vi "Initialize Instrument.vi"(8 "error in (no error)":errorcluster, 10 "Reset":bool, 11 "E3631A in":refnum<class "E3631A.lvclass">) -> (0 "error out":errorcluster, 3 "E3631A out":refnum<class "E3631A.lvclass">)   [LabVIEW 2020, in "E3631A.lvclass"]
uses:
  E3631A.lvclass
  C:/Sandbox/Git_Sandbox/WiSpry Test Framework source code (LV20)/WiSpry Test Framework/Instruments/Instrument.lvclass
  Instrument.lvclass/Instrument.ctl
  Power Supply.lvclass
  Instrument.lvclass
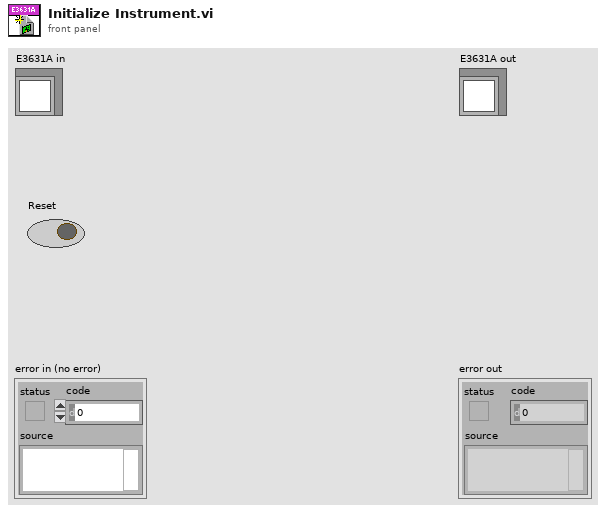
[diagram p1: front panel]
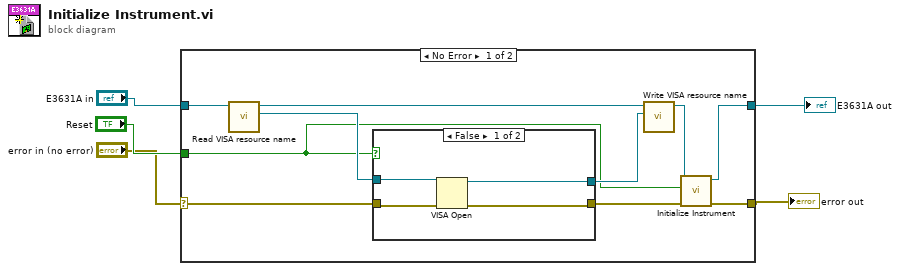
[diagram p0: block diagram]
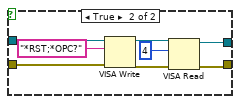
[diagram p2: hidden frame]
diagram:
  n1 = case shown="No Error" "error in (no error)" {
    selector: "error in (no error)" -> [w12 w29]
    tunnel: [w9 w29] -> w1
    tunnel: "E3631A in" -> [w15 w28]
    tunnel: [w7 w28] -> w2
    tunnel: "Reset" -> [w6 _]
    frame No Error {
      n2 = call "Read VISA resource name.vi"("Instrument in"=w15) -> ("VISA resource name"=w13:refnum<visa-resource-name>, "Instrument out"=w14:refnum<class "E3631A.lvclass">)  [unwired: 9 in]
      n3 = case shown="False" w6 {
        tunnel: [w17 w24] -> w10
        tunnel: w13 -> [w18 w27]
        tunnel: w12 -> [w19 w25]
        tunnel: [w16 w20] -> w11
        frame False {
          n4 = VISA Open(error in (no error)=w19, VISA resource name=w18) -> (VISA resource name=w16:refnum<visa-resource-name>, error out=w17:errorcluster)  [unwired: 3 in]
        }
        frame True {
          n5 = VISA Write(VISA resource name=w27, write buffer="*RST;*OPC?", error in (no error)=w25) -> (VISA resource name out=w22:refnum<visa-resource-name>, error out=w23:errorcluster)  [unwired: 1 out]
          n6 = VISA Read(VISA resource name=w22, byte count=u32 4, error in (no error)=w23) -> (VISA resource name out=w20:refnum<visa-resource-name>, error out=w24:errorcluster)  [unwired: 2 out]
        }
      }
      n7 = call "Write VISA resource name.vi"("VISA resource name"=w11, "Instrument in"=w14) -> ("Instrument out"=w8:refnum<class "E3631A.lvclass">)  [unwired: 9 in]
      n8 = call-parent "Initialize Instrument.vi"("error in (no error)"=w10, "Reset"=w6, "Power Supply in"=w8) -> ("error out"=w9:errorcluster, "Power Supply out"=w7:refnum<class "E3631A.lvclass">)  [unwired: 7 in]
    }
    frame Error {
    }
  }
  "error out" <- w1
  "E3631A out" <- w2
